vi "Get Request Type.vi"(8 "error in (no error)":errorcluster, 11 "SetSceneItemEnabled in":refnum<class "SetSceneItemEnabled.lvclass">) -> (0 "error out":errorcluster, 2 "Request Type":string, 3 "SetSceneItemEnabled out":refnum<class "SetSceneItemEnabled.lvclass">)   [LabVIEW 2022 SP3, in "obs-websocket-lv.lvlib" / "SetSceneItemEnabled.lvclass"]
uses:
  SetSceneItemEnabled.lvclass
  SetSceneItemEnabled.lvclass/SetSceneItemEnabled.ctl
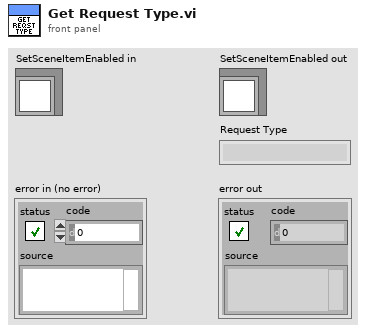
[diagram p1: front panel]
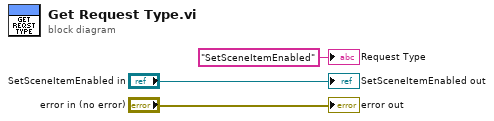
[diagram p0: block diagram]
diagram:
  "error out" <- "error in (no error)"
  "SetSceneItemEnabled out" <- "SetSceneItemEnabled in"
  "Request Type" <- "SetSceneItemEnabled" ("Request Type")
